vi "Flock_Shared_LaunchProcessTemplateVI.vi"(11 "Process List":T1) -> ()   [LabVIEW 2014, in "Flock_Shared_Messaging.lvlib"]
uses:
  Flock_Shared_Messaging.lvlib
  ProcessList.ctl
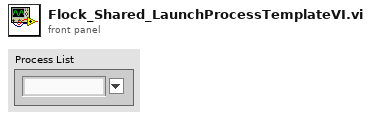
[diagram p1: front panel]
types:
  T1 = typedef "Flock_Shared_Messaging.lvlib/ProcessList.ctl" = string
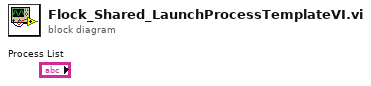
[diagram p0: block diagram]
diagram:
